vi "InitCanByDBCFile.vi"(8 "错误输入":errorcluster, 9 "ASupportedChannelsBased0":string="0", 10 "路径":path=path "D:/安洁资料/B2-EP33L/201017-hd2-EP33L_EP1_WLC-V01.dbc", 11 "CAN_CardProperties":T1={"应用程序名"="APP", "CAN使用通道数"=1, "LIN使用通道数"=0} {"LIN使用通道数" max=5; "CAN使用通道数" min=1 max=1 step=1}) -> (0 "错误输出":errorcluster, 1 "tsdb_load_can_db":i32, 2 "out AId":u32, 3 "应用程序名":string, 5 "ConnectSeccessfully":bool)   [LabVIEW 2016]
uses:
  CAN_Info.ctl
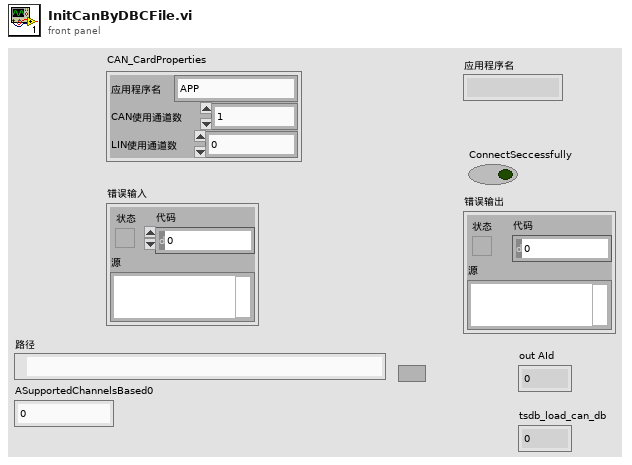
[diagram p1: front panel]
types:
  T1 = typedef "CAN_Info.ctl" = cluster{"应用程序名":string, "CAN使用通道数":u8, "LIN使用通道数":u8}
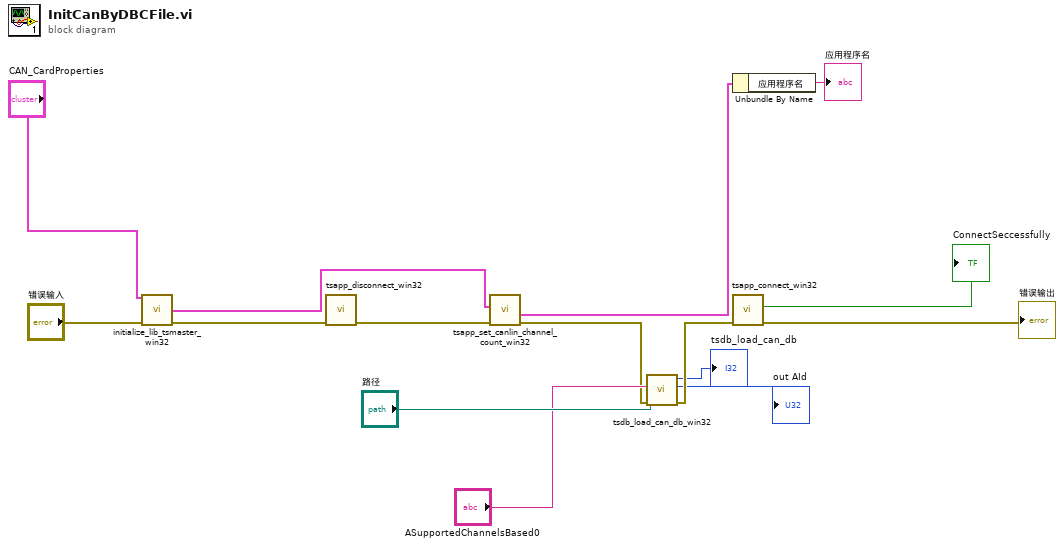
[diagram p0: block diagram]
diagram:
  n1 = call "initialize_lib_tsmaster_win32.vi"("初始化CAN通道"="CAN_CardProperties", "错误输入（无错误）"="错误输入") -> ("InitializationInformation"=w14:T1, "错误输出"=w8:errorcluster)  [unwired: 10 in, 2 out]
  n2 = call "tsapp_disconnect_win32.vi"("错误输入（无错误）"=w8) -> ("错误输出"=w9:errorcluster)  [unwired: 8 in, 2 out]
  n3 = call "tsapp_set_canlin_channel_count_win32.vi"("错误输入（无错误）"=w9, "InitializationInformation"=w14) -> ("错误输出"=w4:errorcluster, "InitializationInformation_Out"=w10:T1)  [unwired: 7 in, 1 out]
  n4 = call "tsdb_load_can_db_win32.vi"("错误输入（无错误）"=w4, "ASupportedChannelsBased0"="ASupportedChannelsBased0", "路径"="路径") -> ("错误输出"=w3:errorcluster, "out AId"=→"out AId":u32, "tsdb_load_can_db"=→"tsdb_load_can_db":i32)  [unwired: 6 in]
  n5 = Unbundle By Name(w10) -> ("应用程序名"=→"应用程序名":string)
  n6 = call "tsapp_connect_win32.vi"("错误输入（无错误）"=w3) -> ("错误输出"=→"错误输出":errorcluster, "ConnectSeccessfully"=→"ConnectSeccessfully":bool)  [unwired: 8 in, 1 out]
